vi "QuickProfile_V4.vi"() -> ()   [LabVIEW 2012]
uses:
  <vilib>/Utility/cursorutil.llb/Set Cursor (Icon Pict).vi
  <vilib>/Utility/file.llb/Write To Spreadsheet File (DBL).vi
panel:
  out "Intensity Graph":sgl[][](graph)
  in  "Select Image":bool
  in  "ROI Size (Pixles)":dbl(slide)=1.0 min=1.0 max=500.0 step=1.0 scale=0.0..100.0 scale format="%#_3g"
  in  "Save ROI":bool
  out "Lorentzian Fit Width (nm)":dbl
  out "Gaussian Fit Width Y (nm)":dbl
  out "Gaussian Fit Width X (nm)":dbl
  in  "Pixel Size (nm)":dbl
  out "Constant Y Slice":cluster{"X Values":dbl[], sgl[]}[](graph)
  out "Constant X Slice":cluster{"X Values":dbl[], sgl[]}[](graph)
  in  "Fit ROI":bool
  out "Gaussian Fit":dbl[][](graph)
  out "Lorentzian Fit":dbl[][](graph)
  out "Current ROI":sgl[][](graph)
  in  "Quit":bool
  # "Constant Y"
  # "Constant X"
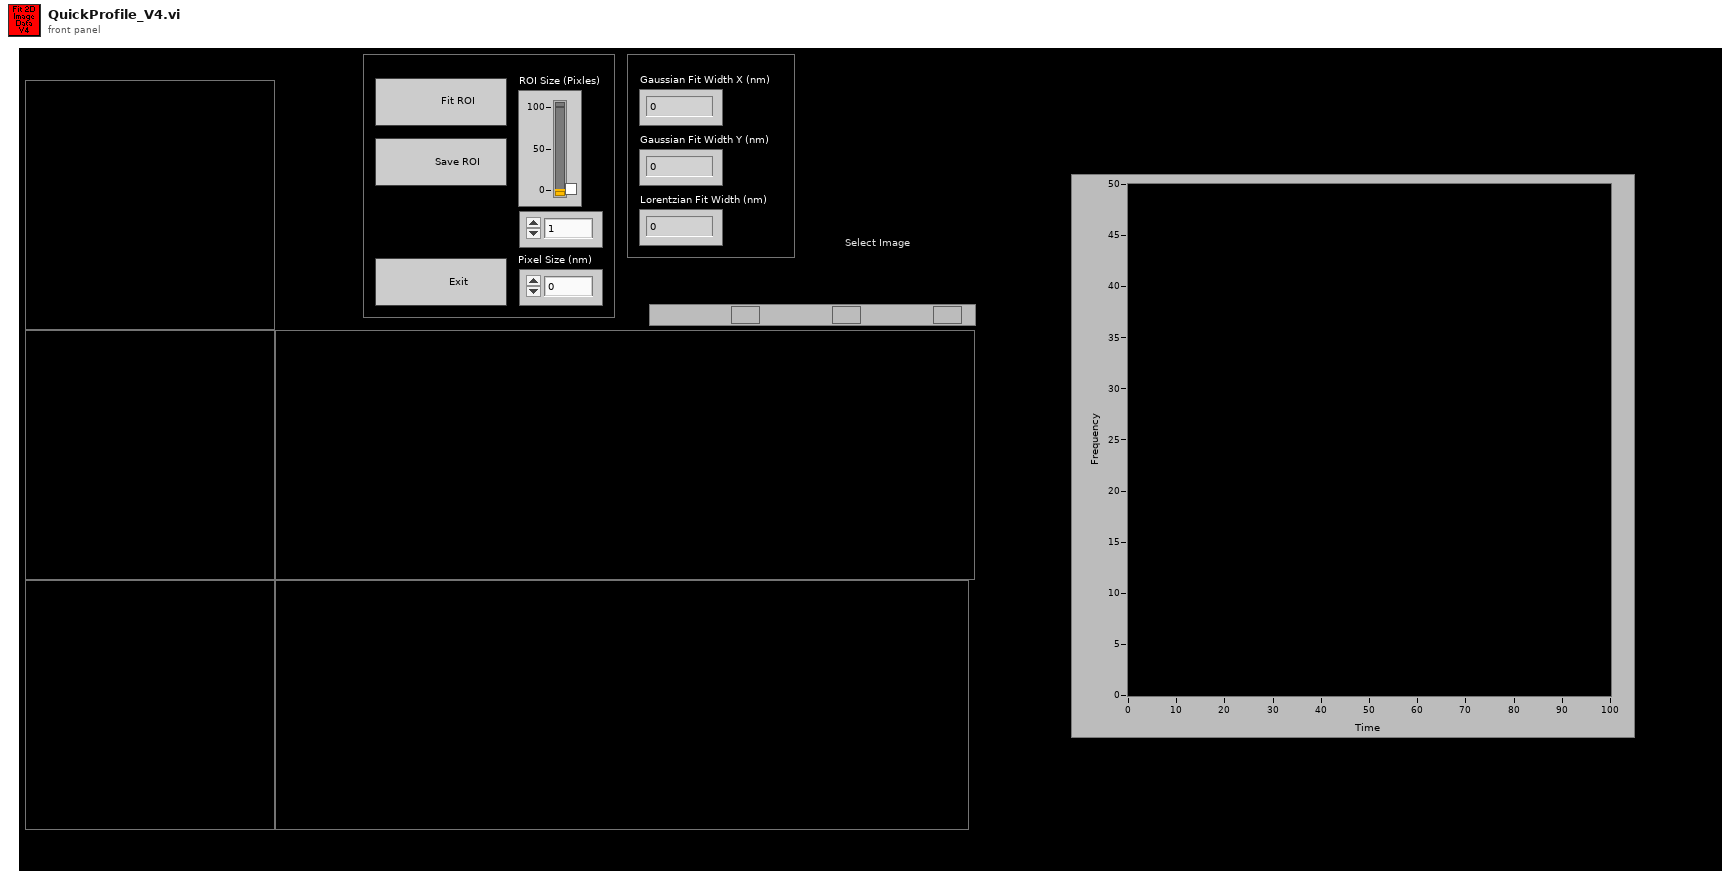
[diagram p1: front panel]
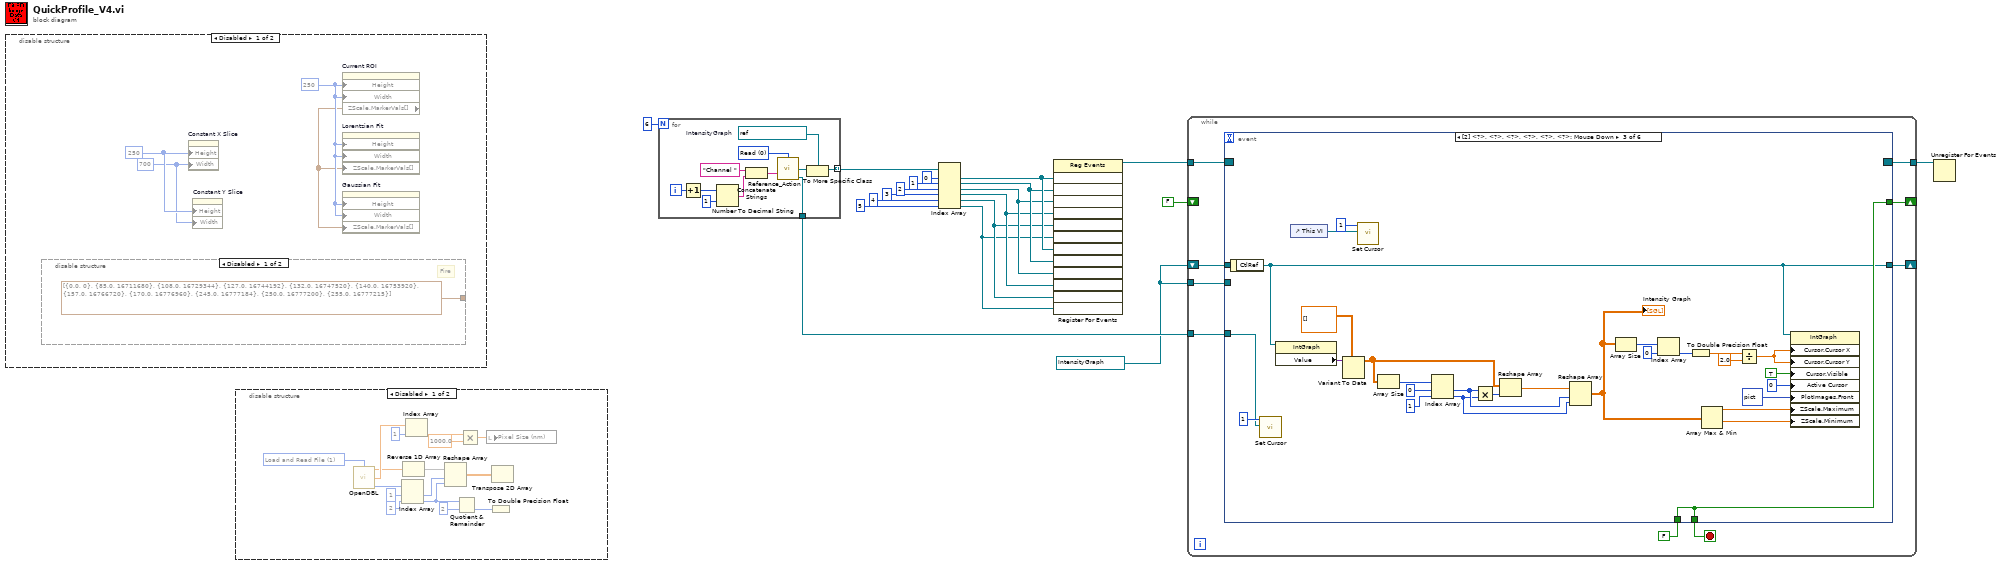
[diagram p0: block diagram]
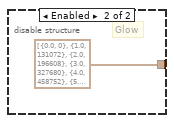
[diagram p3: hidden frame]
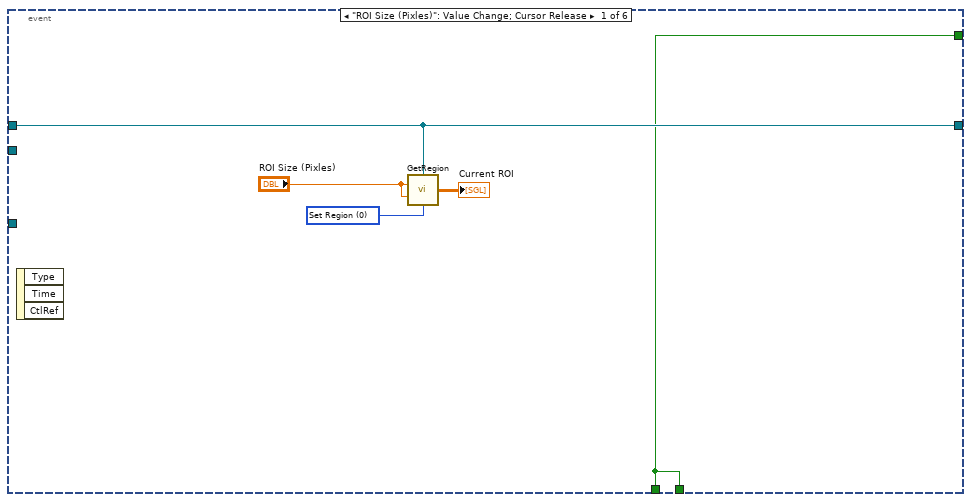
[diagram p5: hidden frame]
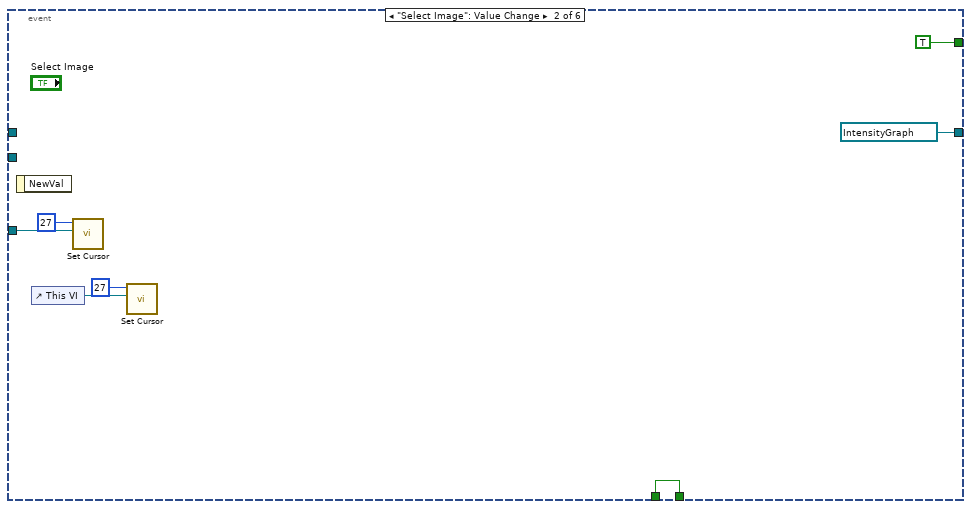
[diagram p6: hidden frame]
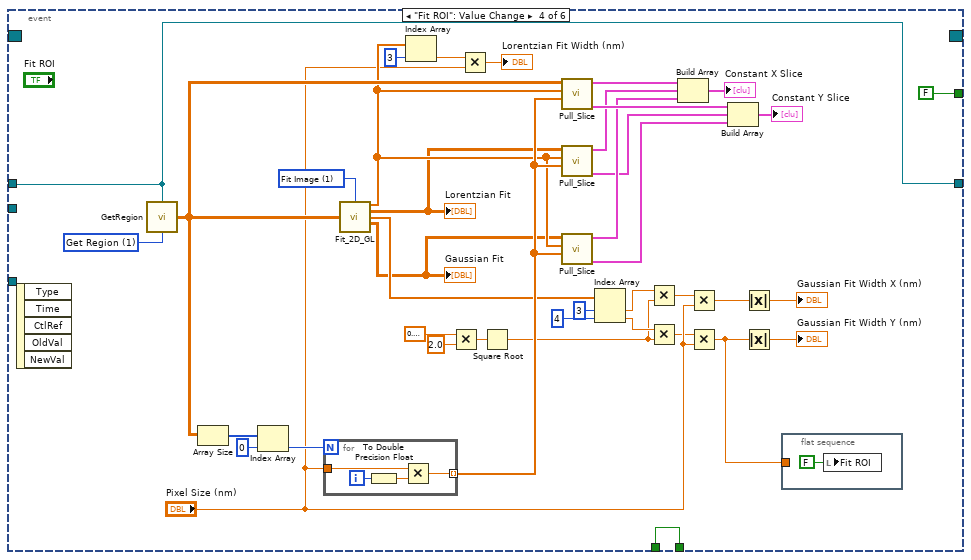
[diagram p7: hidden frame]
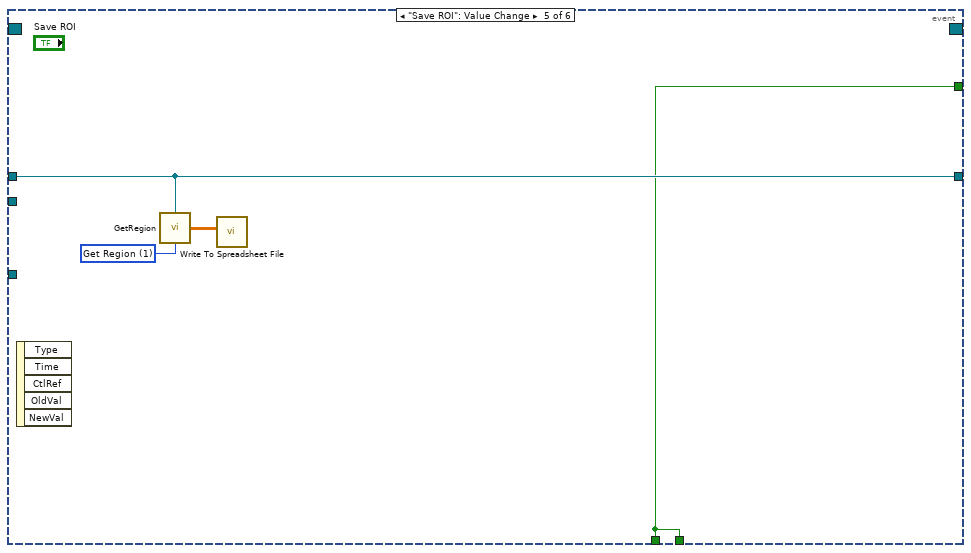
[diagram p8: hidden frame]
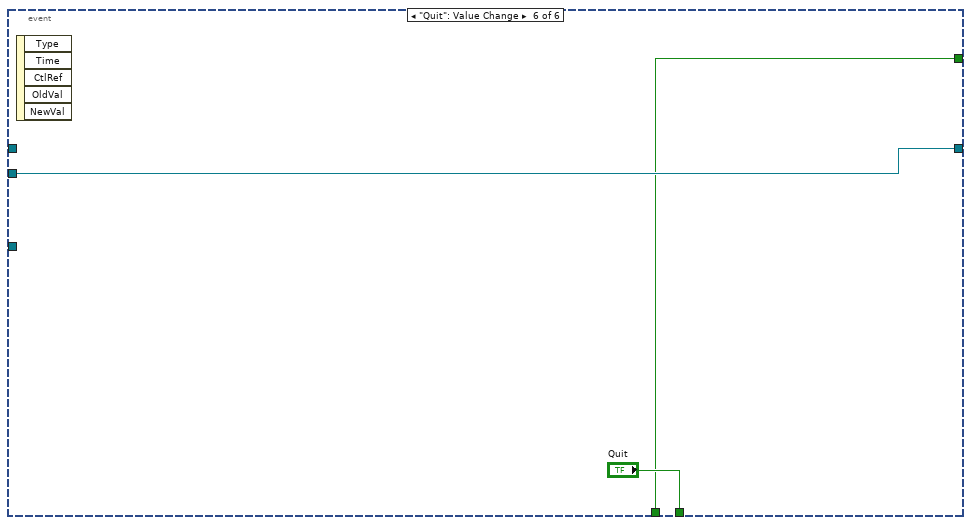
[diagram p9: hidden frame]
diagram:
  w2 = refnum<vi> refnum ("CtlRef")
  n1 = disable-structure shown="Disabled" {
    frame Disabled {
      w21 = u32 700 ("Plot Area:Size:Width")
      w22 = u32 250 ("Plot Area:Size:Height")
      w23 = u32 250 ("Plot Area:Size:Height")
      n2 = disable-structure shown="Disabled" {
        disable-tunnel: [cluster{dbl, u32}[] [{0.0, 0}, {85.0, 16711680}, {108.0, 16729344}, {127.0, 16744192}, {132.0, 16747520}, {140.0, 16753920}, {157.0, 16766720}, {170.0, 16776960}, {245.0, 16777184}, {250.0, 16777200}, {255.0, 16777215}] ("Z Scale.Marker Values[]") cluster{dbl, u32}[] [{0.0, 0}, {1.0, 131072}, {2.0, 196608}, {3.0, 327680}, {4.0, 458752}, {5.0, 589824}, {6.0, 720896}, {7.0, 851971}, {8.0, 983043}, {9.0, 1114115}, {10.0, 1245187}, {11.0, 1376259}, {12.0, 1507331}, {13.0, 1638403}, {14.0, 1769475}, {15.0, 1769479}, {16.0, 2031623}, {17.0, 2162695}, {18.0, 2293767}, {19.0, 2424839}, {20.0, 2555911}, {21.0, 2686983}, {22.0, 2818055}, {23.0, 2949127}, {24.0, 3080203}, {25.0, 3211275}, {26.0, 3342347}, {27.0, 3473419}, {28.0, 3604491}, {29.0, 3735563}, {30.0, 3866635}, {31.0, 3867403}, {32.0, 4129547}, {33.0, 4260619}, {34.0, 4391691}, {35.0, 4522763}, {36.0, 4653839}, {37.0, 4784911}, {38.0, 4915983}, {39.0, 5178127}, {40.0, 5309199}, {41.0, 5440271}, {42.0, 5571343}, {43.0, 5702415}, {44.0, 5703439}, {45.0, 5965583}, {46.0, 6096655}, {47.0, 6227727}, {48.0, 6358799}, {49.0, 6489871}, {50.0, 6620943}, {51.0, 6752015}, {52.0, 6883087}, {53.0, 7015183}, {54.0, 7146255}, {55.0, 7277327}, {56.0, 7408399}, {57.0, 7539471}, {58.0, 7670543}, {59.0, 7801615}, {60.0, 8063759}, {61.0, 8194831}, {62.0, 8326927}, {63.0, 8457999}, {64.0, 8589075}, {65.0, 8720147}, {66.0, 8851219}, {67.0, 8982291}, {68.0, 9113363}, {69.0, 9114387}, {70.0, 9376531}, {71.0, 9507603}, {72.0, 9638675}, {73.0, 9769747}, {74.0, 9901843}, {75.0, 10032915}, {76.0, 10163987}, {77.0, 10229523}, {78.0, 10295059}, {79.0, 10427155}, {80.0, 10558227}, {81.0, 10689299}, {82.0, 10820371}, {83.0, 10886931}, {84.0, 10952467}, {85.0, 11083539}, {86.0, 11214611}, {87.0, 11215635}, {88.0, 11477779}, {89.0, 11543315}, {90.0, 11608851}, {91.0, 11740947}, {92.0, 11806483}, {93.0, 11872019}, {94.0, 12004115}, {95.0, 12135187}, {96.0, 12266259}, {97.0, 12267283}, {98.0, 12398355}, {99.0, 12529427}, {100.0, 12530451}, {101.0, 12595987}, {102.0, 12530451}, {103.0, 12793619}, {104.0, 12794131}, {105.0, 12794643}, {106.0, 13056787}, {107.0, 13057299}, {108.0, 13057811}, {109.0, 13188883}, {110.0, 13320979}, {111.0, 13386515}, {112.0, 13452563}, {113.0, 13584147}, {114.0, 13584659}, {115.0, 13585171}, {116.0, 13585683}, {117.0, 13717267}, {118.0, 13848339}, {119.0, 13849363}, {120.0, 13849875}, {121.0, 13850387}, {122.0, 13981459}, {123.0, 14113555}, {124.0, 14114067}, {125.0, 14114579}, {126.0, 14115091}, {127.0, 14246675}, {128.0, 14377747}, {129.0, 14378771}, {130.0, 14379283}, {131.0, 14379539}, {132.0, 14379795}, {133.0, 14380819}, {134.0, 14511891}, {135.0, 14643987}, {136.0, 14644503}, {137.0, 14645015}, {138.0, 14645527}, {139.0, 14646039}, {140.0, 14646551}, {141.0, 14778135}, {142.0, 14909207}, {143.0, 14910231}, {144.0, 14910747}, {145.0, 14911259}, {146.0, 14911771}, {147.0, 14912283}, {148.0, 14912797}, {149.0, 15044383}, {150.0, 15175455}, {151.0, 15175967}, {152.0, 15176479}, {153.0, 15176991}, {154.0, 15177507}, {155.0, 15178019}, {156.0, 15178531}, {157.0, 15310115}, {158.0, 15441701}, {159.0, 15441959}, {160.0, 15442215}, {161.0, 15442727}, {162.0, 15443243}, {163.0, 15443755}, {164.0, 15444269}, {165.0, 15444783}, {166.0, 15444783}, {167.0, 15576367}, {168.0, 15707953}, {169.0, 15708467}, {170.0, 15708979}, {171.0, 15708981}, {172.0, 15708983}, {173.0, 15710011}, {174.0, 15710523}, {175.0, 15711037}, {176.0, 15711039}, {177.0, 15711553}, {178.0, 15843139}, {179.0, 15974213}, {180.0, 15974215}, {181.0, 15974217}, {182.0, 15974219}, {183.0, 15975755}, {184.0, 15976271}, {185.0, 15976785}, {186.0, 15977299}, {187.0, 15977301}, {188.0, 15977815}, {189.0, 15978327}, {190.0, 15978331}, {191.0, 16109917}, {192.0, 16241503}, {193.0, 16241505}, {194.0, 16242019}, {195.0, 16242535}, {196.0, 16242537}, {197.0, 16242539}, {198.0, 16243563}, {199.0, 16243567}, {200.0, 16244081}, {201.0, 16244595}, {202.0, 16244599}, {203.0, 16244601}, {204.0, 16244603}, {205.0, 16245627}, {206.0, 16245631}, {207.0, 16245633}, {208.0, 16246147}, {209.0, 16246663}, {210.0, 16377735}, {211.0, 16508811}, {212.0, 16508815}, {213.0, 16509839}, {214.0, 16509843}, {215.0, 16509845}, {216.0, 16509847}, {217.0, 16510361}, {218.0, 16510875}, {219.0, 16510879}, {220.0, 16510881}, {221.0, 16510883}, {222.0, 16511399}, {223.0, 16511911}, {224.0, 16511915}, {225.0, 16511917}, {226.0, 16511919}, {227.0, 16511923}, {228.0, 16512437}, {229.0, 16512951}, {230.0, 16512955}, {231.0, 16512957}, {232.0, 16512959}, {233.0, 16512961}, {234.0, 16512963}, {235.0, 16512967}, {236.0, 16513481}, {237.0, 16513995}, {238.0, 16513999}, {239.0, 16514001}, {240.0, 16514003}, {241.0, 16514005}, {242.0, 16514007}, {243.0, 16514011}, {244.0, 16514013}, {245.0, 16514015}, {246.0, 16514019}, {247.0, 16514021}, {248.0, 16514023}, {249.0, 16514027}, {250.0, 16514029}, {251.0, 16514031}, {252.0, 16514035}, {253.0, 16514037}, {254.0, 16514039}, {255.0, 16514043}] ("Z Scale.Marker Values[]")] -> _
        frame Disabled {
          # "Fire"
        }
        frame Enabled {
          # "Glow"
        }
      }
      n3 = property on="Constant X Slice" class="XYGraph (strict)"("Height"=w22, "Width"=w21) -> ()  [unwired: 2 in, 2 out]
      n4 = property on="Constant Y Slice" class="XYGraph (strict)"("Height"=w22, "Width"=w21) -> ()  [unwired: 2 in, 2 out]
      n5 = property on="Current ROI" class="IntGraph (strict)"("Height"=w23, "Width"=w23) -> ("ZScale.MarkerVals[]"=w20:cluster{dbl, u32}[])  [unwired: 2 in, 2 out]
      n6 = property on="Lorentzian Fit" class="IntGraph (strict)"("Height"=w23, "Width"=w23, "ZScale.MarkerVals[]"=w20) -> ()  [unwired: 2 in, 2 out]
      n7 = property on="Gaussian Fit" class="IntGraph (strict)"("Height"=w23, "Width"=w23, "ZScale.MarkerVals[]"=w20) -> ()  [unwired: 2 in, 2 out]
    }
    frame Enabled {
    }
  }
  n8 = disable-structure shown="Disabled" {
    frame Disabled {
      w26 = u16 1 items=["Get Image", "Load and Read File"] ("Action")
      n9 = call "OpenDBL.vi"("Action"=w26) -> ("Image"=w27:sgl[], "Physical Length (Z, Y, X, t)"=w33:sgl[], "Dimensions (Z, Y, X, t)"=w28:i32[])  [unwired: 11 in, 1 out]
      n10 = Index Array(array=w28, index #1=1 ("index"), index #2=2 ("index")) -> (element #1=w31:i32, element #2=w38:i32)
      n11 = Reverse 1D Array(array=w27) -> (reversed array=w41:sgl[])
      n12 = Index Array(array=w33, index=1) -> (element=w35:sgl)
      n13 = Reshape Array(w41, w31, w38) -> (w32:sgl[][])
      n14 = Quotient & Remainder(x=w38, y=2) -> (floor(x/y)=w40:i32)  [unwired: 1 out]
      n15 = Multiply(x=w35, y=sgl 1000.0) -> (x*y=w37:sgl)
      n16 = local write "Pixel Size (nm)"(w37) -> ()
      n17 = To Double Precision Float(number=w40) -> ()  [unwired: 1 out]
      n18 = Transpose 2D Array(2D array=w32) -> ()  [unwired: 1 out]
    }
    frame Enabled {
    }
  }
  n19 = for {
    N: 6 -> [_]
    tunnel: [w44] -> w13 mode=indexing
    tunnel: [w42] -> w4
    i -> [w51]
    w48 = u16 0 items=["Read", "Initialize"] ("Action")
    w46 = refnum<vi> refnum  # IntensityGraph
    n20 = Increment(x=w51) -> (x+1=w43:i32)
    n21 = Number To Decimal String(number=w43, width (-)=i16 1) -> (decimal integer string=w50:string)
    n22 = Concatenate Strings("Channel " ("string"), w50) -> (w45:string)
    n23 = call "Reference_Action.vi"("Action"=w48, "Control Name"=w45) -> ("Ref OUT"=w47:refnum<vi>, "VI Reference"=w42:refnum<vi>)  [unwired: 12 in]
    n24 = To More Specific Class(target class=w46, reference=w47) -> (specific class reference=w44:refnum<vi>)  [unwired: 1 in, 1 out]
  }
  n25 = Index Array(array=w13, index #1=0 ("index"), index #2=1 ("index"), index #3=2 ("index"), index #4=3 ("index"), index #5=4 ("index"), index #6=5 ("index")) -> (element #1=w10:refnum<vi>, element #2=w9:refnum<vi>, element #3=w8:refnum<vi>, element #4=w7:refnum<vi>, element #5=w6:refnum<vi>, element #6=w5:refnum<vi>)
  n26 = register-events(w10, w9, w8, w7, w6, w5, w10, w9, w8, w7, w6, w5) -> (reference out=w11:refnum<event-registration>)  [unwired: 2 in, 1 out]
  n27 = while {
    tunnel: w11 -> [w59]
    tunnel: w4 -> [w58]
    shift-right: [w57] -> _
    shift-left: FALSE -> [_]
    shift-right: [w56] -> _
    shift-left: w2 -> [w55]
    tunnel: w2 -> [w54]
    tunnel: [w53] -> w1
    stop <- w61 stop-if-true
    n28 = event shown="[2] <?>, <?>, <?>, <?>, <?>, <?>: Mouse Down" {
      selector: w59 -> [_ _ _ _ _ _]
      dyn-events: [_ _ _ _ _ _] -> w53
      timeout: _ -> [_ _ _ _ _ _]
      tunnel: [w62 w69 w101 w141 w147 "Quit"] -> w61
      tunnel: FALSE -> [w62 w69 w101 w141 w147 w151]
      tunnel: w58 -> [_ w70 w77 _ _ _]
      tunnel: [w62 TRUE w101 FALSE w147 w151] -> w57
      tunnel: [w63 refnum<vi> refnum ("CtlRef") w87 w103 w148 w152] -> w56
      tunnel: w55 -> [w63 _ _ w103 w148 _]
      tunnel: w54 -> [_ _ _ _ _ w152]
      event "ROI Size (Pixles)": Value Change; Cursor Release {
        w66 = u16 0 items=["Set Region", "Get Region"] ("Action")
        n29 = event-data() -> ()  [unwired: 1 in, 3 out]
        n30 = call "GetRegion.vi"("IntGraph REF"=w63, "Y Width (PX)"="ROI Size (Pixles)", "X Width (PX)"="ROI Size (Pixles)", "Action"=w66) -> ("Region Out"=→"Current ROI":sgl[][])  [unwired: 11 in]
      }
      event "Select Image": Value Change {
        n31 = event-data() -> ()  [unwired: 1 in, 1 out]
        n32 = control-ref of="This VI"() -> (w73:refnum<vi>)
        n33 = call-poly <vilib>:"Set Cursor.vi"("VI reference (current VI)"=w70, "icon"=u16 27) -> ()  [unwired: 8 in, 2 out]
        n34 = call-poly <vilib>:"Set Cursor.vi"("VI reference (current VI)"=w73, "icon"=u16 27) -> ()  [unwired: 8 in, 2 out]
      }
      event Mouse Down {
        n35 = event-data() -> ("CtlRef"=w87:refnum<vi>)  [unwired: 1 in]
        n36 = call-poly <vilib>:"Set Cursor.vi"("VI reference (current VI)"=w77, "icon"=u16 1) -> ()  [unwired: 8 in, 2 out]
        n37 = property class="IntGraph"(reference=w87) -> ("Value"=w100:variant)  [unwired: 1 in, 2 out]
        n38 = control-ref of="This VI"() -> (w78:refnum<vi>)
        n39 = Variant To Data(type=sgl[][] [], Variant=w100) -> (data=w75:sgl[][])  [unwired: 1 in, 1 out]
        n40 = call-poly <vilib>:"Set Cursor.vi"("VI reference (current VI)"=w78, "icon"=u16 1) -> ()  [unwired: 8 in, 2 out]
        n41 = Array Size(array=w75) -> (size(s)=w93:i32[])
        n42 = Index Array(array=w93, index #1=0 ("index"), index #2=1 ("index")) -> (element #1=w98:i32, element #2=w97:i32)
        n43 = Multiply(x=w98, y=w97) -> (x*y=w95:i32)
        n44 = Reshape Array(w75, w95) -> (w74:sgl[])
        n45 = Reshape Array(w74, w98, w97) -> (w76:sgl[][])
        "Intensity Graph" <- w76
        n46 = Array Size(array=w76) -> (size(s)=w88:i32[])
        n47 = Index Array(array=w88, index=0) -> (element=w90:i32)
        n48 = To Double Precision Float(number=w90) -> (double precision float=w92:dbl)
        n49 = Array Max & Min(array=w76) -> (max value=w82:sgl, min value=w81:sgl)  [unwired: 2 out]
        n50 = Divide(x=w92, y=2.0) -> (x/y=w86:dbl)
        n51 = property class="IntGraph"(reference=w87, "Cursor.Cursor X"=w86, "Cursor.Cursor Y"=w86, "Cursor.Visible"=TRUE, "Active Cursor"=u32 0, "PlotImages.Front"=picture data[5B] ("Plot Images:Front"), "ZScale.Maximum"=w82, "ZScale.Minimum"=w81) -> ()  [unwired: 1 in, 2 out]
      }
      event "Fit ROI": Value Change {
        w139 = u16 1 items=["Read Fit Data", "Fit Image"] ("Action")
        w140 = u16 1 items=["Set Region", "Get Region"] ("Action")
        n52 = event-data() -> ()  [unwired: 1 in, 5 out]
        n53 = call "GetRegion.vi"("IntGraph REF"=w103, "Action"=w140) -> ("Region Out"=w129:sgl[][])  [unwired: 13 in]
        n54 = Array Size(array=w129) -> (size(s)=w138:i32[])
        n55 = Index Array(array=w138, index=0) -> (element=w136:i32)
        n56 = for {
          N: w136 -> [_]
          tunnel: "Pixel Size (nm)" -> [w145]
          tunnel: [w143] -> w135 mode=indexing
          i -> [w146]
          n57 = To Double Precision Float(number=w146) -> (double precision float=w144:dbl)
          n58 = Multiply(x=w145, y=w144) -> (x*y=w143:dbl)
        }
        n59 = call "Fit_2D_GL.vi"("Action"=w139, "Image IN"=w129) -> ("Lorentz Fit Parameters"=w124:dbl[], "Lorentzian Image"=w115:dbl[][], "Gaussian Fit Parameters"=w126:dbl[], "Gaussian Image"=w114:dbl[][])  [unwired: 10 in]
        "Gaussian Fit" <- w114
        "Lorentzian Fit" <- w115
        n60 = Index Array(array=w124, index=3) -> (element=w120:dbl)
        n61 = Multiply(x=0.6931471805599453, y=2.0) -> (x*y=w109:dbl)
        n62 = Multiply(x=w120, y="Pixel Size (nm)") -> (x*y=→"Lorentzian Fit Width (nm)":dbl)
        n63 = Square Root(x=w109) -> (sqrt(x)=w106:dbl)
        n64 = call "Pull_Slice.vi"("X Values"=w135, "Fit Parameters"=w124, "ROI Image"=w129) -> ("Constant X Slice"=w134:cluster{"X Values":dbl[], sgl[]}, "Constant Y Slice"=w121:cluster{"X Values":dbl[], sgl[]})  [unwired: 7 in]
        n65 = call "Pull_Slice.vi"("X Values"=w135, "Fit Parameters"=w124, "ROI Image"=w115) -> ("Constant X Slice"=w131:cluster{"X Values":dbl[], sgl[]}, "Constant Y Slice"=w133:cluster{"X Values":dbl[], sgl[]})  [unwired: 7 in]
        n66 = call "Pull_Slice.vi"("X Values"=w135, "Fit Parameters"=w124, "ROI Image"=w114) -> ("Constant X Slice"=w130:cluster{"X Values":dbl[], sgl[]}, "Constant Y Slice"=w132:cluster{"X Values":dbl[], sgl[]})  [unwired: 7 in]
        n67 = Index Array(array=w126, index #1=3 ("index"), index #2=4 ("index")) -> (element #1=w113:dbl, element #2=w111:dbl)
        n68 = Multiply(x=w113, y=w106) -> (x*y=w112:dbl)
        n69 = Multiply(x=w111, y=w106) -> (x*y=w110:dbl)
        n70 = Build Array(w121, w133, w132) -> (→"Constant X Slice":cluster{"X Values":dbl[], sgl[]}[])
        n71 = Multiply(x=w112, y="Pixel Size (nm)") -> (x*y=w118:dbl)
        n72 = Multiply(x=w110, y="Pixel Size (nm)") -> (x*y=w116:dbl)
        n73 = Build Array(w134, w131, w130) -> (→"Constant Y Slice":cluster{"X Values":dbl[], sgl[]}[])
        n74 = Absolute Value(x=w118) -> (abs(x)=→"Gaussian Fit Width X (nm)":dbl)
        n75 = Absolute Value(x=w116) -> (abs(x)=→"Gaussian Fit Width Y (nm)":dbl)
        n76 = flat-sequence {
          tunnel: w116 -> [_]
          frame #0 {
            n77 = local write "Fit ROI"(FALSE ("Fit ROI")) -> ()
          }
        }
      }
      event "Save ROI": Value Change {
        w150 = u16 1 items=["Set Region", "Get Region"] ("Action")
        n78 = event-data() -> ()  [unwired: 1 in, 5 out]
        n79 = call "GetRegion.vi"("IntGraph REF"=w148, "Action"=w150) -> ("Region Out"=w149:sgl[][])  [unwired: 13 in]
        n80 = call-poly <vilib>:"Write To Spreadsheet File.vi"("2D data"=w149) -> ()  [unwired: 7 in, 1 out]
      }
      event "Quit": Value Change {
        n81 = event-data() -> ()  [unwired: 1 in, 5 out]
      }
    }
  }
  n82 = Unregister For Events(event registration refnum=w1) -> ()  [unwired: 1 in, 1 out]
